vi "Distancia Global.vi"() -> ()   [LabVIEW 2014]
panel:
  out "Distancia":dbl
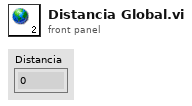
[diagram p1: front panel]
diagram:
